vi "Initialize Parameter File.vi"(6 "File type":enum16{"INI"}(ring), 8 "error in (no error)":errorcluster, 9 "create file if necessary (T)":bool=TRUE, 10 "configuration file path (blank opens dialog)":path, 11 "CD Parameter Manager in":refnum<class "CD Parameter Manager.lvclass">) -> (0 "error out":errorcluster, 2 "Cancelled?":bool, 3 "CD Parameter Manager out":refnum<class "CD Parameter Manager.lvclass">)   [LabVIEW 2019, in "CD Parameter Manager API.lvlib" / "CD Parameter Manager.lvclass"]
uses:
  CD Parameter Manager.lvclass
  Parameter INI File/Parameter INI File.lvclass
  C:/Repositories/CSD_Custom_Device/CSD_Custom_Device/Source/Libraries/CD Parameter Manager API/Parameter Generic File/Parameter Generic File.lvclass
  CD Parameter Manager.lvclass/CD Parameter Manager.ctl
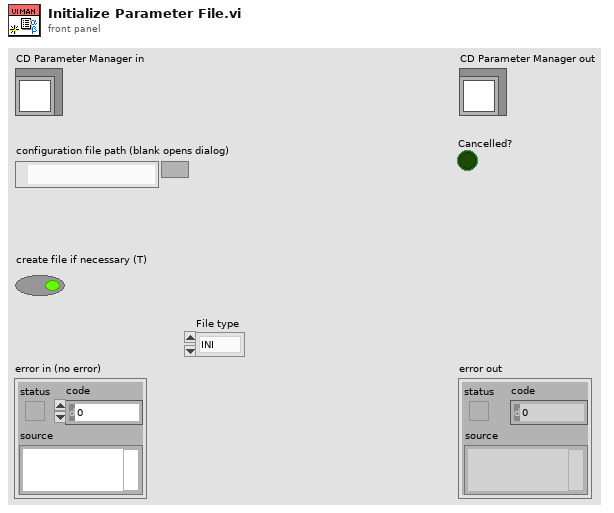
[diagram p1: front panel]
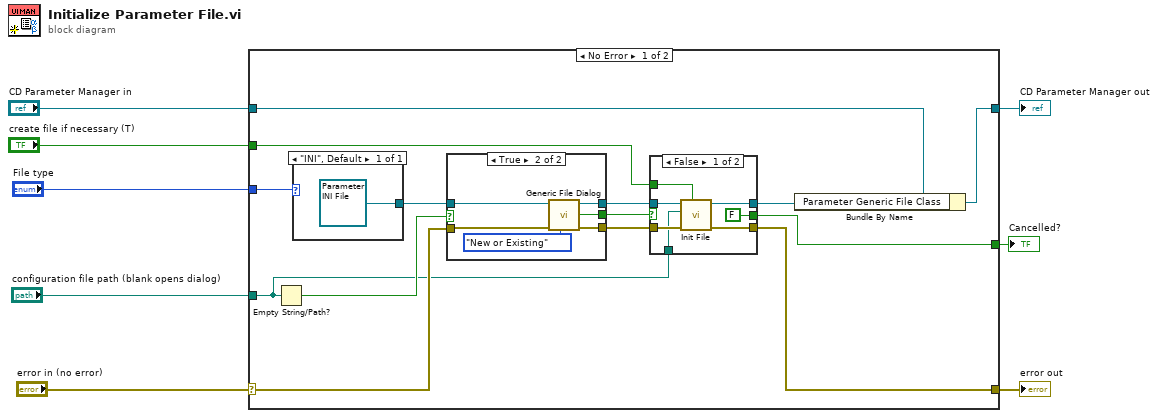
[diagram p0: block diagram]
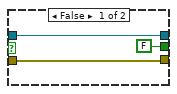
[diagram p3: hidden frame]
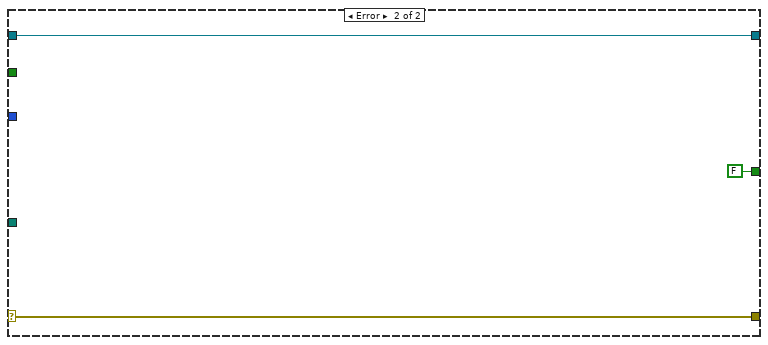
[diagram p4: hidden frame]
diagram:
  n1 = case shown="No Error" "error in (no error)" {
    selector: "error in (no error)" -> [w18 w45]
    tunnel: [w14 w45] -> w7
    tunnel: [w12 w44] -> w5
    tunnel: "CD Parameter Manager in" -> [w17 w44]
    tunnel: "File type" -> [w22 _]
    tunnel: "configuration file path (blank opens dialog)" -> [w11 _]
    tunnel: "create file if necessary (T)" -> [w13 _]
    tunnel: [w9 FALSE] -> w1
    frame No Error {
      n2 = Empty String/Path?(string/path=w11) -> (empty?=w21:bool)
      n3 = case shown="\"INI\", Default" w22 {
        tunnel: [refnum<class "Parameter INI File.lvclass"> refnum ("CD Parameter Manager API.lvlib:Parameter INI File.lvclass")] -> w20
        frame "INI", Default {
        }
      }
      n4 = case shown="True" w21 {
        tunnel: w20 -> [w35 w41]
        tunnel: [w35 w40] -> w19
        tunnel: w18 -> [w34 w39]
        tunnel: [w34 w38] -> w15
        tunnel: [FALSE ("Cancelled?") w36] -> w10
        frame False {
        }
        frame True {
          n5 = call-dynamic "Generic File Dialog.vi"("Selection mode"=enum16{"New", "Existing", "New or Existing"}."New or Existing", "error in (no error)"=w39, "Parameter INI File in"=w41) -> ("error out"=w38:errorcluster, "Cancelled?"=w36:bool, "Parameter INI File out"=w40:refnum<class "Parameter INI File.lvclass">)  [unwired: 6 in]
        }
      }
      n6 = case shown="False" w10 {
        selector: w10 -> [_ w30]
        tunnel: w19 -> [w29 w32]
        tunnel: [w28 w32] -> w16
        tunnel: w15 -> [w27 w31]
        tunnel: [w26 w31] -> w14
        tunnel: w13 -> [w25 _]
        tunnel: w11 -> [w24 _]
        tunnel: [FALSE w30] -> w9
        frame False {
          n7 = call-dynamic "Init File.vi"("create file if necessary (T)"=w25, "error in (no error)"=w27, "configuration file path"=w24, "Parameter INI File in"=w29) -> ("error out"=w26:errorcluster, "Parameter INI File out"=w28:refnum<class "Parameter INI File.lvclass">)  [unwired: 6 in]
        }
        frame True {
        }
      }
      n8 = Bundle By Name(cluster=w17, "Parameter Generic File Class"=w16) -> (w12:refnum<class "CD Parameter Manager.lvclass">)
    }
    frame Error {
    }
  }
  "error out" <- w7
  "CD Parameter Manager out" <- w5
  "Cancelled?" <- w1
